vi "Dispose.vi"(8 "error in (no error)":errorcluster, 11 "Pointer in":refnum<class "Pointer.lvclass">) -> (0 "error out":errorcluster, 3 "Pointer out":refnum<class "Pointer.lvclass">)   [LabVIEW 2016, in "Memory Manager.lvlib" / "Pointer.lvclass"]
doc: "Disposes of the provided <b>pointer</b> and deallocates the associated memory."
uses:
  Pointer.lvclass
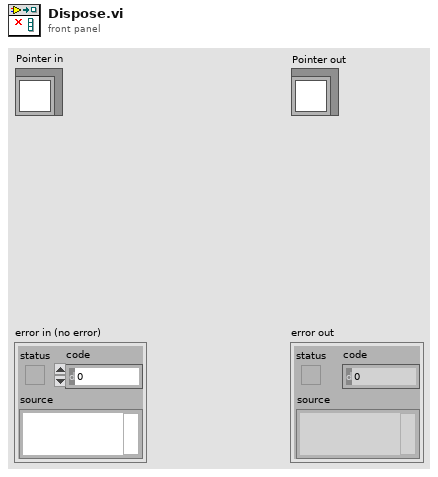
[diagram p1: front panel]
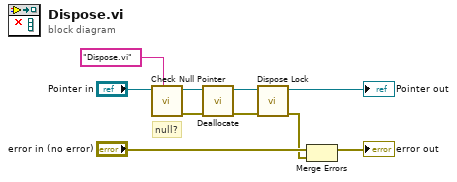
[diagram p0: block diagram]
diagram:
  # "null?"
  n1 = call "Check Null Pointer.vi"("source vi name"="Dispose.vi", "Pointer in"="Pointer in") -> ("error out"=w7:errorcluster, "Pointer out"=w8:refnum<class "Pointer.lvclass">)  [unwired: 8 in]
  n2 = call "Deallocate.vi"("error in (no error)"=w7, "Pointer in"=w8) -> ("error out"=w3:errorcluster, "Pointer out"=w4:refnum<class "Pointer.lvclass">)  [unwired: 8 in]
  n3 = call-dynamic "Dispose Lock.vi"("error in (no error)"=w3, "Pointer in"=w4) -> ("error out"=w2:errorcluster, "Pointer out"=→"Pointer out":refnum<class "Pointer.lvclass">)  [unwired: 8 in]
  n4 = Merge Errors("error in (no error)", w2) -> (→"error out":errorcluster)
